vi "hmp4000 Initialize with Options.vi"(0 "VISA resource name":refnum<visa-resource-name>, 2 "Option string (\"\")":string, 5 "ID Query (T: Check)":bool=TRUE, 7 "Reset (T: Reset)":bool=TRUE, 11 "error in (no error)":errorcluster) -> (4 "VISA resource name out":refnum<visa-resource-name>, 15 "error out":errorcluster)   [LabVIEW 2022 SP3]
doc: "This VI opens a new session to the instrument.\nCompared to the <b>Initialize.vi</b>, this one allows for additional settings in the <b>Option string</b>."
uses:
  type_Session_Parameter_int32.ctl
  type_InterfaceType.ctl
  type_Session_Parameter_Boolean.ctl
  type_AdditionalFlag_Bits.ctl
  hmp4000_core_global.vi
  hmp4000_rsidr_core.lvlib
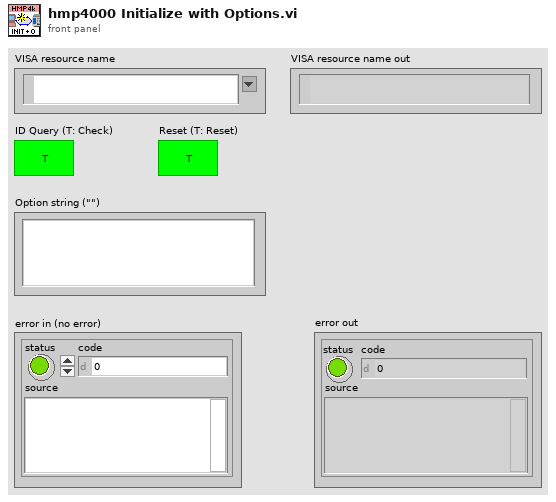
[diagram p1: front panel]
types:
  T1 = typedef "hmp4000_rsidr_core.lvlib/type_AdditionalFlag_Bits.ctl" = enum16{"Send LF after Bin Block", "Junk read with io_clear_buffers.vi", "io_clear_buffers: viClear()", "io_clear_buffers: viFlush()", "<NotUsed1>", "Allow Dbl & Int Bin/Ascii read", "*OPC? in check_instrument_error.vi", "<NotUsed2>", "Smart Enum Matching", "Less Strict RepCaps check", "AssureResponseEndWithLF"}
  T2 = typedef "hmp4000_rsidr_core.lvlib/type_Session_Parameter_Boolean.ctl" = enum16{"Simulate", "Query Instr Status", "Check Range", "Check Options", "Add LF to Write", "Duplicate Session", "Fast Sweep", "Logging"}
  T3 = typedef "hmp4000_rsidr_core.lvlib/type_Session_Parameter_int32.ctl" = enum16{"OPC Timeout", "Additional Flags", "Wait Before Write", "Wait Before Read", "Bin Data Chunk Size", "VISA Access Mode", "VISA Timeout", "Bin Float Number Format", "Bin Integer Number Format", "STBpollVISAtimeout", "OPCwaitMode"}
  T4 = typedef "hmp4000_rsidr_core.lvlib/type_InterfaceType.ctl" = enum16{"Unknown", "GPIB", "VXI", "GPIB_VXI", "ASRL", "PXI", "TCPIP", "USB", "SOCKET"}
  T5 = typedef "hmp4000_rsidr_core.lvlib/type_Input_Format_RepCap.ctl" = cluster{"repCapName":string, "indetifiers":string[], "cmdValues":string[]}
  T6 = typedef "hmp4000_rsidr_core.lvlib/type_Input_Format_RangeTable.ctl" = cluster{"Type":u16, "Name":string, "Entries":cluster{"Name":string, "Value 1":dbl, "Value 2":dbl, "Command":string}[]}
  T7 = typedef "hmp4000_rsidr_core.lvlib/type_Input_Format_Attribute.ctl" = cluster{"Level":i32, "Class Only":bool, "Identifier":string, "Descriptive Name":string, "Data Type":u16, "Command":string, "Access":u16, "Range Table":string, "Read Callback":string, "Write Callback":string, "Supported Models":string, "Instrument Options":string, "Flags":i32, "Help":string}
  T8 = typedef "hmp4000_rsidr_core.lvlib/type_Session_Data.ctl" = cluster{"IDN string":string, "Instrument FW":string, "Instr type":string, "Instr type for err. msg.":string, "Installed Options":string[], "Ignore Error Messages":string, "Logging params":variant, "OPC Timeout":i32, "VISA Timeout":i32, "STB Poll VISA Timeout":i32, "Additional Flags":i32, "Wait Before Read":i32, "Wait Before Write":i32, "Option String Flags":i32, "IO Segment Size":i64, "VISA Access Mode":T9, "Interface Type":T4, "OPC Wait Mode":T10, "Bin Float Number  Format":T11, "Bin Integer Number Format":T12, "Simulate":bool, "VXIcapable":bool, "Duplicate Session":bool, "Add LF to Write":bool, "Logging":bool, "Fast Sweep":bool, "Query Instrument Status":bool, "Check Range":bool, "Check Options":bool}
  T9 = typedef "hmp4000_rsidr_core.lvlib/type_VisaAccessMode.ctl" = u16
  T10 = typedef "hmp4000_rsidr_core.lvlib/type_OPC_Wait_Mode.ctl" = enum16{"STBpolling", "STBpollingSlow", "STBpollingSuperSlow", "ServiceRequest", "OPCquery"}
  T11 = typedef "hmp4000_rsidr_core.lvlib/type_Binary_Float_Number_Format.ctl" = enum16{"Float_4_Bytes_Swapped", "Float_4_Bytes", "Double_8_Bytes_Swapped", "Double_8_Bytes"}
  T12 = typedef "hmp4000_rsidr_core.lvlib/type_Binary_Integer_Number_Format.ctl" = enum16{"Int32_4_Bytes_Swapped", "Int32_4 Bytes", "Int16_2_Bytes_Swapped", "Int16_2_Bytes"}
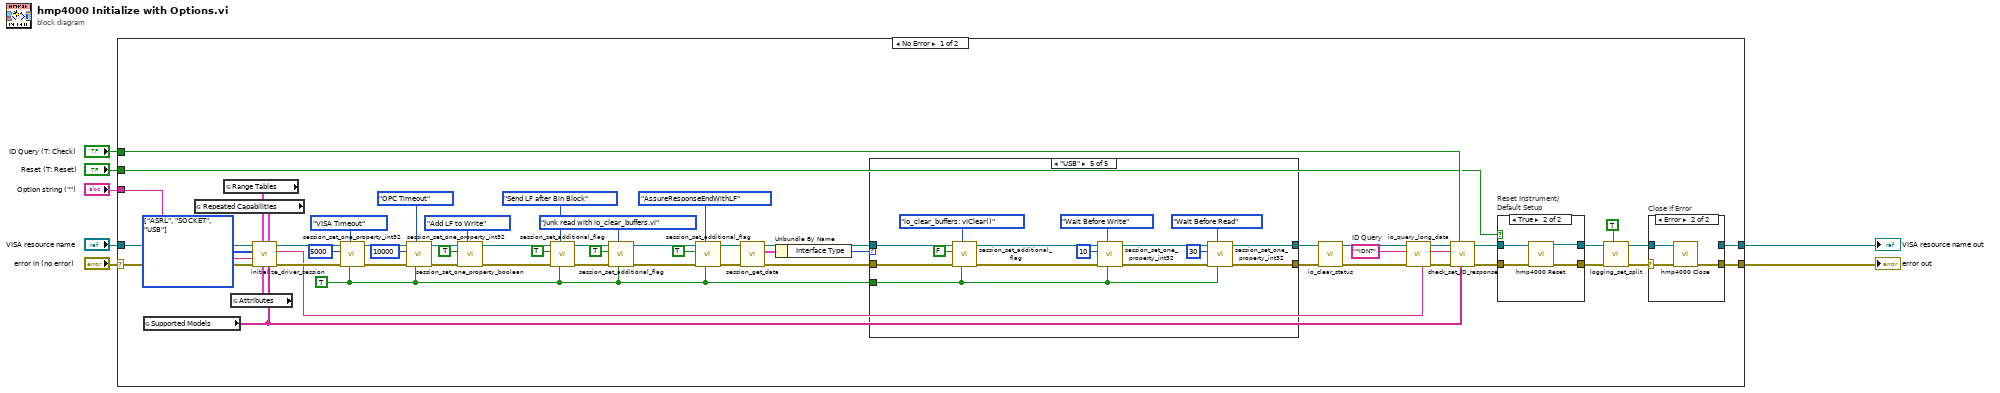
[diagram p0: block diagram]
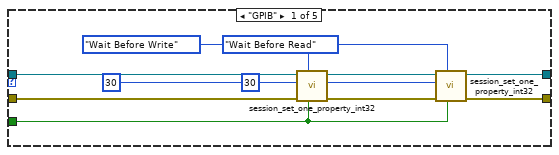
[diagram p2: hidden frame]
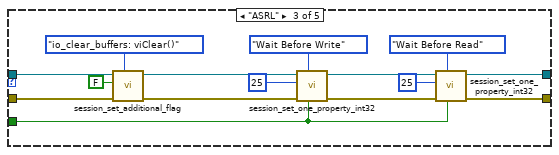
[diagram p4: hidden frame]
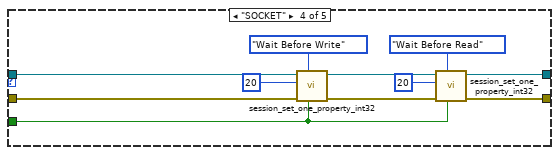
[diagram p5: hidden frame]
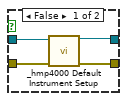
[diagram p7: hidden frame]
diagram:
  n1 = case shown="No Error" "error in (no error)" {
    selector: "error in (no error)" -> [w62 w134]
    tunnel: [w66 _] -> w7
    tunnel: [w63 w134] -> w6
    tunnel: "VISA resource name" -> [w61 _]
    tunnel: "ID Query (T: Check)" -> [w55 _]
    tunnel: "Reset (T: Reset)" -> [w54 _]
    tunnel: "Option string (\"\")" -> [w53 _]
    frame No Error {
      w13 = TRUE ("Skip setting if in Options string (F)")
      w46 = T4[] [enum."ASRL", enum."SOCKET", enum."USB"] items=["Unknown", "GPIB", "VXI", "GPIB_VXI", "ASRL", "PXI", "TCPIP", "USB", "SOCKET"] ("Non-VXI sessions list (\"ASRL,SOCKET\")")
      w21 = "*IDN?"  # ID Query
      n2 = global read "hmp4000_core_global.vi" "Supported Models"() -> (w50:string[])
      n3 = global read "hmp4000_core_global.vi" "Repeated Capabilities"() -> (w47:T5[])
      n4 = global read "hmp4000_core_global.vi" "Range Tables"() -> (w52:T6[])
      n5 = global read "hmp4000_core_global.vi" "Attributes"() -> (w51:T7[])
      n6 = call "initialize_driver_session.vi"("Supported instruments"=w50, "Repeated Capabilities"=w47, "Attributes"=w51, "Range Tables"=w52, "error in"=w62, "Option String"=w53, "Non-VXI sessions list (\"ASRL,SOCKET\")"=w46, "VISA resource name"=w61) -> ("error out"=w45:errorcluster, "Simulation *IDN? response out"=w20:string, "VISA resource name out"=w44:refnum<visa-resource-name>)  [unwired: 1 in]
      n7 = call "session_set_one_property_int32.vi"("Skip setting if in Options string (F)"=w13, "Session Parameter Integer"=type_Session_Parameter_int32."VISA Timeout", "error in"=w45, "Int32 value in"=5000, "VISA resource name"=w44) -> ("error out"=w43:errorcluster, "VISA resource name out"=w42:refnum<visa-resource-name>)  [unwired: 4 in, 1 out]
      n8 = call "session_set_one_property_int32.vi"("Skip setting if in Options string (F)"=w13, "Session Parameter Integer"=type_Session_Parameter_int32."OPC Timeout", "error in"=w43, "Int32 value in"=10000, "VISA resource name"=w42) -> ("error out"=w39:errorcluster, "VISA resource name out"=w38:refnum<visa-resource-name>)  [unwired: 4 in, 1 out]
      n9 = call "session_set_one_property_boolean.vi"("Session Parameter Boolean"=type_Session_Parameter_Boolean."Add LF to Write", "error in"=w39, "Boolean value in"=TRUE, "VISA resource name"=w38) -> ("error out"=w35:errorcluster, "VISA resource name out"=w34:refnum<visa-resource-name>)  [unwired: 5 in, 1 out]
      n10 = call "session_set_additional_flag.vi"("Skip setting if in Options string (F)"=w13, "AdditionalFlag Bit"=type_AdditionalFlag_Bits."Send LF after Bin Block", "error in"=w35, "New value in"=TRUE, "VISA resource name"=w34) -> ("error out"=w29:errorcluster, "VISA resource name out"=w28:refnum<visa-resource-name>)  [unwired: 4 in, 1 out]
      n11 = call "session_set_additional_flag.vi"("Skip setting if in Options string (F)"=w13, "AdditionalFlag Bit"=type_AdditionalFlag_Bits."Junk read with io_clear_buffers.vi", "error in"=w29, "New value in"=TRUE, "VISA resource name"=w28) -> ("error out"=w25:errorcluster, "VISA resource name out"=w24:refnum<visa-resource-name>)  [unwired: 4 in, 1 out]
      n12 = call "session_set_additional_flag.vi"("Skip setting if in Options string (F)"=w13, "AdditionalFlag Bit"=type_AdditionalFlag_Bits."AssureResponseEndWithLF", "error in"=w25, "New value in"=TRUE, "VISA resource name"=w24) -> ("error out"=w17:errorcluster, "VISA resource name out"=w16:refnum<visa-resource-name>)  [unwired: 4 in, 1 out]
      n13 = call "session_get_data.vi"("error in"=w17, "VISA resource name"=w16) -> ("error out"=w12:errorcluster, "Session User Data out"=w15:T8, "VISA resource name out"=w11:refnum<visa-resource-name>)  [unwired: 6 in, 1 out]
      n14 = Unbundle By Name(w15) -> ("Interface Type"=w14:T4)
      n15 = case shown="\"USB\"" w14 {
        tunnel: w13 -> [w75 _ w92 w103 w106]
        tunnel: w12 -> [w74 w79 w83 w102 w114]
        tunnel: w11 -> [w73 w78 w82 w101 w113]
        tunnel: [w70 w79 w89 w98 w108] -> w10
        tunnel: [w69 w78 w88 w97 w107] -> w9
        frame "GPIB" {
          n16 = call "session_set_one_property_int32.vi"("Skip setting if in Options string (F)"=w75, "Session Parameter Integer"=type_Session_Parameter_int32."Wait Before Write", "error in"=w74, "Int32 value in"=30, "VISA resource name"=w73) -> ("error out"=w72:errorcluster, "VISA resource name out"=w71:refnum<visa-resource-name>)  [unwired: 4 in, 1 out]
          n17 = call "session_set_one_property_int32.vi"("Skip setting if in Options string (F)"=w75, "Session Parameter Integer"=type_Session_Parameter_int32."Wait Before Read", "error in"=w72, "Int32 value in"=30, "VISA resource name"=w71) -> ("error out"=w70:errorcluster, "VISA resource name out"=w69:refnum<visa-resource-name>)  [unwired: 4 in, 1 out]
        }
        frame Default {
        }
        frame "ASRL" {
          n18 = call "session_set_additional_flag.vi"("AdditionalFlag Bit"=type_AdditionalFlag_Bits."io_clear_buffers: viClear()", "error in"=w83, "New value in"=FALSE, "VISA resource name"=w82) -> ("error out"=w81:errorcluster, "VISA resource name out"=w80:refnum<visa-resource-name>)  [unwired: 5 in, 1 out]
          n19 = call "session_set_one_property_int32.vi"("Skip setting if in Options string (F)"=w92, "Session Parameter Integer"=type_Session_Parameter_int32."Wait Before Write", "error in"=w81, "Int32 value in"=25, "VISA resource name"=w80) -> ("error out"=w91:errorcluster, "VISA resource name out"=w90:refnum<visa-resource-name>)  [unwired: 4 in, 1 out]
          n20 = call "session_set_one_property_int32.vi"("Skip setting if in Options string (F)"=w92, "Session Parameter Integer"=type_Session_Parameter_int32."Wait Before Read", "error in"=w91, "Int32 value in"=25, "VISA resource name"=w90) -> ("error out"=w89:errorcluster, "VISA resource name out"=w88:refnum<visa-resource-name>)  [unwired: 4 in, 1 out]
        }
        frame "SOCKET" {
          n21 = call "session_set_one_property_int32.vi"("Skip setting if in Options string (F)"=w103, "Session Parameter Integer"=type_Session_Parameter_int32."Wait Before Write", "error in"=w102, "Int32 value in"=20, "VISA resource name"=w101) -> ("error out"=w100:errorcluster, "VISA resource name out"=w99:refnum<visa-resource-name>)  [unwired: 4 in, 1 out]
          n22 = call "session_set_one_property_int32.vi"("Skip setting if in Options string (F)"=w103, "Session Parameter Integer"=type_Session_Parameter_int32."Wait Before Read", "error in"=w100, "Int32 value in"=20, "VISA resource name"=w99) -> ("error out"=w98:errorcluster, "VISA resource name out"=w97:refnum<visa-resource-name>)  [unwired: 4 in, 1 out]
        }
        frame "USB" {
          n23 = call "session_set_additional_flag.vi"("Skip setting if in Options string (F)"=w106, "AdditionalFlag Bit"=type_AdditionalFlag_Bits."io_clear_buffers: viClear()", "error in"=w114, "New value in"=FALSE, "VISA resource name"=w113) -> ("error out"=w112:errorcluster, "VISA resource name out"=w111:refnum<visa-resource-name>)  [unwired: 4 in, 1 out]
          n24 = call "session_set_one_property_int32.vi"("Skip setting if in Options string (F)"=w106, "Session Parameter Integer"=type_Session_Parameter_int32."Wait Before Write", "error in"=w112, "Int32 value in"=10, "VISA resource name"=w111) -> ("error out"=w110:errorcluster, "VISA resource name out"=w109:refnum<visa-resource-name>)  [unwired: 4 in, 1 out]
          n25 = call "session_set_one_property_int32.vi"("Skip setting if in Options string (F)"=w106, "Session Parameter Integer"=type_Session_Parameter_int32."Wait Before Read", "error in"=w110, "Int32 value in"=30, "VISA resource name"=w109) -> ("error out"=w108:errorcluster, "VISA resource name out"=w107:refnum<visa-resource-name>)  [unwired: 4 in, 1 out]
        }
      }
      n26 = call "io_clear_status.vi"("error in"=w10, "VISA resource name"=w9) -> ("error out"=w23:errorcluster, "VISA resource name out"=w22:refnum<visa-resource-name>)  [unwired: 8 in]
      n27 = call "io_query_long_data.vi"("Simulation read buffer (\"Simulation\")"=w20, "error in"=w23, "write buffer"=w21, "VISA resource name"=w22) -> ("error out"=w19:errorcluster, "read buffer"=w8:string, "VISA resource name out"=w18:refnum<visa-resource-name>)  [unwired: 5 in]
      n28 = call "check_set_ID_response.vi"("Supported instruments in"=w50, "Error if ID Query check fails"=w55, "error in"=w19, "IDN string in"=w8, "VISA resource name"=w18) -> ("error out"=w64:errorcluster, "VISA resource name out"=w65:refnum<visa-resource-name>)  [unwired: 3 in, 2 out]
      n29 = case "Reset Instrument/\nDefault Setup" shown="True" w54 {
        tunnel: w64 -> [w129 w133]
        tunnel: [w128 w132] -> w60
        tunnel: w65 -> [w127 w131]
        tunnel: [w126 w130] -> w59
        frame False {
          n30 = call "_hmp4000 Default Instrument Setup.vi"("VISA resource name"=w127, "error in (no error)"=w129) -> ("VISA resource name out"=w126:refnum<visa-resource-name>, "error out"=w128:errorcluster)  [unwired: 12 in]
        }
        frame True {
          n31 = call "hmp4000 Reset.vi"("VISA resource name"=w131, "error in (no error)"=w133) -> ("VISA resource name out"=w130:refnum<visa-resource-name>, "error out"=w132:errorcluster)  [unwired: 12 in]
        }
      }
      n32 = call "logging_set_split.vi"("Evaluate section error (F)"=TRUE, "error in"=w60, "VISA resource name"=w59) -> ("error out"=w58:errorcluster, "VISA resource name out"=w57:refnum<visa-resource-name>)  [unwired: 7 in]
      n33 = case "Close if Error" shown="Error" w58 {
        selector: w58 -> [w121 w124]
        tunnel: w57 -> [w122 w125]
        tunnel: [w122 _] -> w66
        tunnel: [w121 w123] -> w63
        frame No Error {
        }
        frame Error {
          n34 = call "hmp4000 Close.vi"("error in (no error)"=w124, "VISA resource name"=w125) -> ("error out"=w123:errorcluster)  [unwired: 9 in]
        }
      }
    }
    frame Error {
    }
  }
  "VISA resource name out" <- w7
  "error out" <- w6
